vi "HMI.vi"(8 "error in (no error)":errorcluster caption="entrée d'erreur (pas d'erreur)", 11 "Popup Operator_Input Batch In":refnum<class "Class Popup Operator_Input SN.lvclass">) -> (0 "error out":errorcluster caption="sortie d'erreur", 1 "Input":string="Attente \nvalidation", 2 "Operator_Selection":bool, 3 "Popup Operator_Input Batch In":refnum<class "Class Popup Operator_Input SN.lvclass">)   [LabVIEW 2020, in "Library Instrument & Equipement.lvlib" / "Library Popup.lvlib" / "Class Popup Operator_Input SN.lvclass"]
uses:
  Class Popup Operator_Input SN.lvclass
  C:/Users/ngarcin/OneDrive - Altyor/Standard TB/Class/Popup/Class Popup (Main)/Class Popup (Main).lvclass
  JSON API/JSON Value/Set from JSON string.vi
  JSON API/JSON Value/JSON Value.lvclass
  Class Popup (Main)/Class Popup (Main).lvclass
  Class Popup Operator_Input SN.lvclass/Class Popup Operator_Input SN.ctl
  JSON API/Variant JSON/Variant JSON.lvlib
  JSON API/Get Polymorphic/JSON GetSet.lvlib
panel:
  in  "Bouton NOK":bool
  in  "Input OP":string="Attente \nvalidation"
  in  "Bouton OK":bool
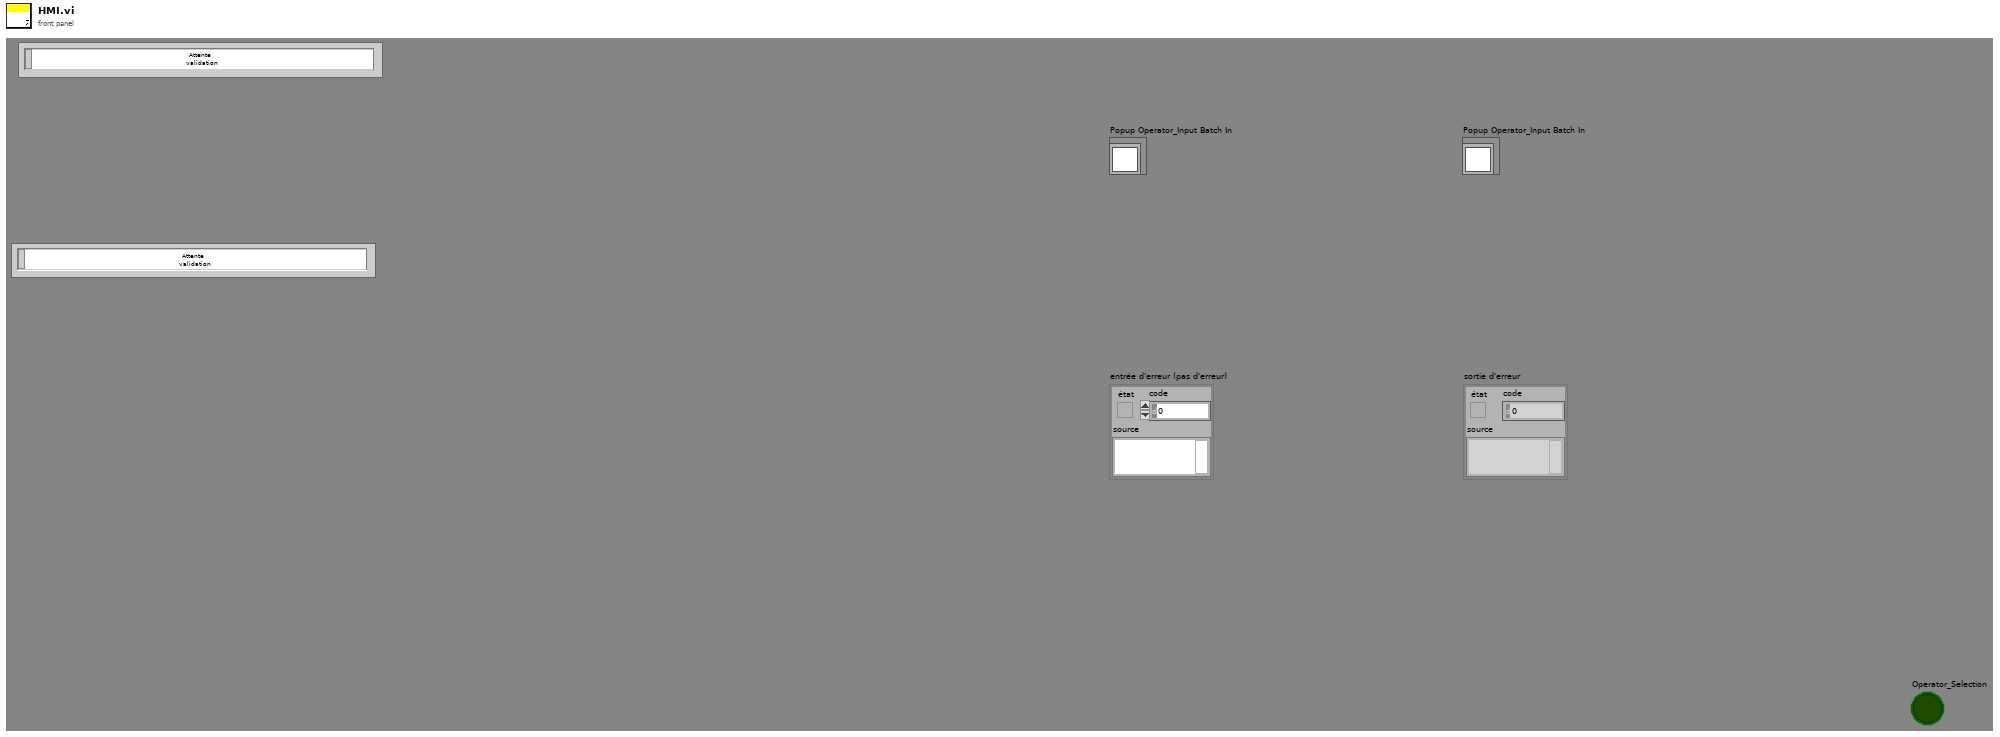
[diagram p1: front panel]
types:
  T1 = enum32{"Invalid", "Standard", "Closed", "Hidden", "Minimized", "Maximized"}
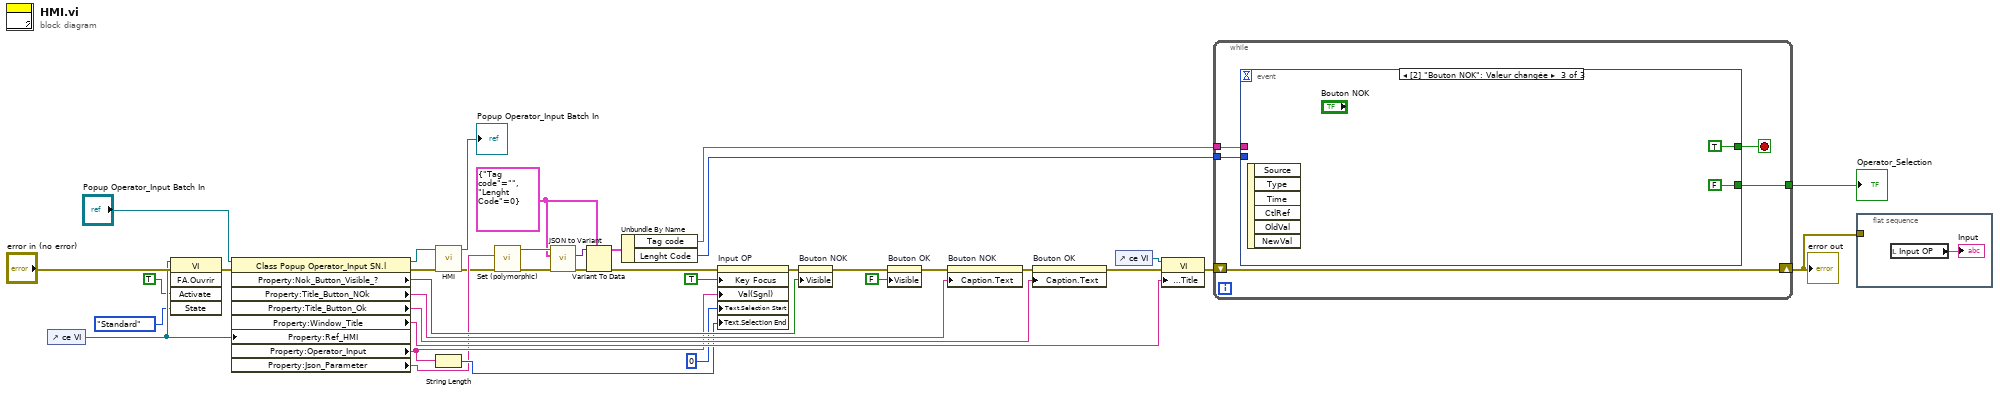
[diagram p0: block diagram]
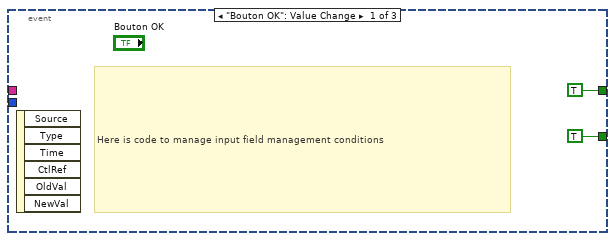
[diagram p2: hidden frame]
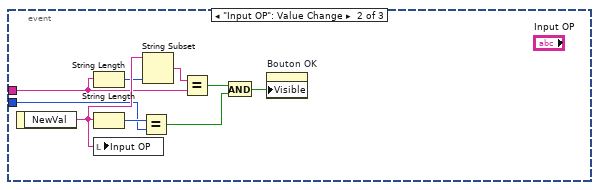
[diagram p3: hidden frame]
diagram:
  w12 = cluster{"Tag code":string, "Lenght Code":i32} {"Tag code"="", "Lenght Code"=0}
  n1 = control-ref of="ce VI"() -> (w7:refnum<vi>)
  n2 = invoke class="VI" method="FA.Ouvrir"(reference=w7, error in="error in (no error)", "Activate"=TRUE ("Fenêtre face-avant:Au premier plan"), "State"=T1."Standard" ("État")) -> (error out=w6:errorcluster)  [unwired: 1 in, 4 out]
  n3 = property class="Class Popup Operator_Input SN.l"(reference="Popup Operator_Input Batch In", error in=w6, "Property:Ref_HMI"=w7) -> (reference out=w33:refnum<class "Class Popup Operator_Input SN.lvclass">, error out=w2:errorcluster, "Property:Nok_Button_Visible_?"=w38:bool, "Property:Title_Button_NOk"=w32:string, "Property:Title_Button_Ok"=w30:string, "Property:Window_Title"=w35:string, "Property:Operator_Input"=w22:string, "Property:Json_Parameter"=w14:string)
  n4 = call-parent "HMI.vi"("error in (no error)"=w2, "Class Popup (Main) en entrée"=w33) -> ("error out"=w1:errorcluster, "Class Popup (Main) en sortie"=→"Popup Operator_Input Batch In":refnum<class "Class Popup Operator_Input SN.lvclass">)  [unwired: 6 in, 2 out]
  n5 = String Length(string=w22) -> (length=w24:i32)
  n6 = call-poly "Set (polymorphic).vi"("error in (no error)"=w1, "JSON stream"=w14) -> ("error out"=w16:errorcluster, "JSON Value out"=w18:refnum<class "JSON Value.lvclass">)  [unwired: 7 in, 1 out]
  n7 = call "JSON to Variant.vi"("error in (no error)"=w16, "Variant (Data Type)"=w12, "JSON Value"=w18) -> ("error out"=w17:errorcluster, "Variant out"=w15:variant)  [unwired: 7 in]
  n8 = Variant To Data(error in=w17, type=w12, Variant=w15) -> (data=w11:cluster{"Tag code":string, "Lenght Code":i32}, error out=w13:errorcluster)
  n9 = Unbundle By Name(w11) -> ("Tag code"=w10:string, "Lenght Code"=w9:i32)
  n10 = property on="Input OP" class="Ch"(error in=w13, "Key Focus"=TRUE ("Focus clavier"), "Val(Sgnl)"=w22, "Text.Selection Start"=u32 0 ("Texte.Sélection:Début"), "Text.Selection End"=w24) -> (error out=w3:errorcluster)  [unwired: 1 in, 1 out]
  n11 = property on="Bouton NOK" class="Bool"(error in=w3, "Visible"=w38) -> (error out=w28:errorcluster)  [unwired: 1 in, 1 out]
  n12 = property on="Bouton OK" class="Bool"(error in=w28, "Visible"=FALSE ("Activer ?")) -> (error out=w27:errorcluster)  [unwired: 1 in, 1 out]
  n13 = property on="Bouton NOK" class="Bool"(error in=w27, "Caption.Text"=w32) -> (error out=w31:errorcluster)  [unwired: 1 in, 1 out]
  n14 = property on="Bouton OK" class="Bool"(error in=w31, "Caption.Text"=w30) -> (error out=w25:errorcluster)  [unwired: 1 in, 1 out]
  n15 = control-ref of="ce VI"() -> (w36:refnum<vi>)
  n16 = property class="VI"(reference=w36, error in=w25, "Front Panel.Title"=w35) -> (error out=w34:errorcluster)  [unwired: 1 out]
  n17 = while {
    tunnel: [w41] -> w37
    shift-right: [w42] -> w21
    shift-left: w34 -> [w42]
    tunnel: w10 -> [w40]
    tunnel: w9 -> [w39]
    stop <- w43 stop-if-true
    n18 = event shown="[2] \"Bouton NOK\": Valeur changée" {
      selector: _ -> [_ _ _]
      dyn-events: _ -> [_ _ _]
      timeout: _ -> [_ _ _]
      tunnel: [TRUE ("Valeur (Signalisation)") _ TRUE ("Valeur (Signalisation)")] -> w43
      tunnel: [TRUE ("Operator_Selection") _ FALSE ("Operator_Selection")] -> w41
      tunnel: w40 -> [_ w48 _]
      tunnel: w39 -> [_ w46 _]
      event "Bouton OK": Value Change {
        # "Here is code to manage input field management conditions"
        n19 = event-data() -> ()  [unwired: 1 in, 6 out]
      }
      event "Input OP": Value Change {
        n20 = event-data() -> ("NewVal"=w49:string)  [unwired: 1 in]
        n21 = String Length(string=w48) -> (length=w47:i32)
        n22 = String Length(string=w49) -> (length=w52:i32)
        n23 = local write "Input OP"(w49) -> ()
        n24 = Equal?(x=w52, y=w46) -> (x = y?=w51:bool)
        n25 = String Subset(string=w49, length (rest)=w47) -> (substring=w54:string)  [unwired: 1 in]
        n26 = Equal?(x=w54, y=w48) -> (x = y?=w53:bool)
        n27 = And(x=w53, y=w51) -> (x .and. y?=w50:bool)
        n28 = property on="Bouton OK" class="Bool"("Visible"=w50) -> ()  [unwired: 2 in, 2 out]
      }
      event "Bouton NOK": Value Change {
        n29 = event-data() -> ()  [unwired: 1 in, 6 out]
      }
    }
  }
  "error out" <- w21
  "Operator_Selection" <- w37
  n30 = flat-sequence {
    tunnel: w21 -> [_]
    frame #0 {
      n31 = local read "Input OP"() -> (→"Input":string)
    }
  }
